vi "Setup_variables.vi"(3 "setup":T1) -> ()   [LabVIEW 2010]
uses:
  Controls/Setup.ctl
  Globals/Meas_global.vi
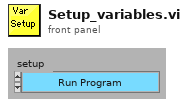
[diagram p1: front panel]
types:
  T1 = typedef "Setup.ctl" = enum16{"Run Program", "Show Setup", "Save Current Setup", "Setup Front Panel"}
  T2 = typedef "Ch_and_Spans.ctl" = cluster{"high limit (10V)":sgl, "low limit (-10V)":sgl, "Ch No":i16, "Var name":string, "Use Latest Calib":bool}
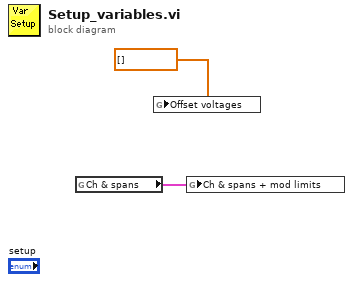
[diagram p0: block diagram]
diagram:
  n1 = global read "Meas_global.vi" "Ch & spans"() -> (w1:T2[])
  n2 = global write "Meas_global.vi" "Offset voltages"(dbl[] [] ("Offset voltages used")) -> ()
  n3 = global write "Meas_global.vi" "Ch & spans + mod limits"(w1) -> ()
